vi "Close Apps.vi"(1 "error in":errorcluster) -> (0 "error out":errorcluster)   [LabVIEW 2015, in "AguaClara Library.lvlib"]
uses:
  AguaClara Library.lvlib
  AutoCAD cmds.ctl
  Word cmd.ctl
  Mathcad Prime cmds.ctl
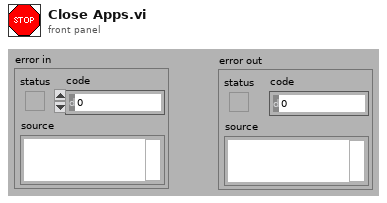
[diagram p1: front panel]
types:
  T1 = typedef "Mathcad Prime cmds.ctl" = enum16{"Open Mathcad", "Open Worksheet", "Send Inputs", "Read Results", "Quit Mathcad"}
  T2 = typedef "AguaClara Library.lvlib/Word cmd.ctl" = enum16{"Initialize", "Load User Inputs", "Update Fields", "Replace Variables", "Save pdf", "Close Word"}
  T3 = typedef "AguaClara Library.lvlib/AutoCAD cmds.ctl" = enum16{"Open AutoCAD", "New Document", "Send Command", "Send Command Array", "Close Doc", "Quit"}
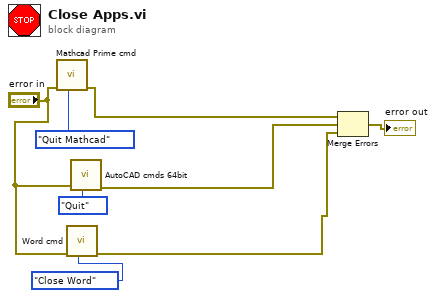
[diagram p0: block diagram]
diagram:
  n1 = call "Mathcad Prime cmd.vi"("Mathcad Prime cmds"=Mathcad_Prime_cmds."Quit Mathcad", "error in (no error)"="error in") -> ("error out"=w4:errorcluster)  [unwired: 7 in, 2 out]
  n2 = call "Word cmd.vi"("Word cmd"=Word_cmd."Close Word", "Error In (no error)"="error in") -> ("error out"=w2:errorcluster)  [unwired: 8 in, 1 out]
  n3 = call "AutoCAD cmds 64bit.vi"("AutoCAD cmd"=AutoCAD_cmds."Quit", "error in (no error)"="error in") -> ("error out"=w3:errorcluster)  [unwired: 7 in, 2 out]
  n4 = Merge Errors(w4, w3, w2) -> (→"error out":errorcluster)
